vi "Configure Trigger (State).vi"(0 "VISA resource name":refnum<visa-resource-name>, 1 "State Condition (0: AND)":i32(ring) items=["And", "Not And"], 5 "Trigger Source (1: Channel1)":i32(ring)=1 items=["Channel1"=1, "Channel2"=2, "Channel3"=3, "Channel4"=4, "DIG0"=20, "DIG1"=21, "DIG2"=22, "DIG3"=23, "DIG4"=24, "DIG5"=25, "DIG6"=26, "DIG7"=27, "DIG8"=28, "DIG9"=29, "DIG10"=30, "DIG11"=31, "DIG12"=32, "DIG13"=33, "DIG14"=34, "DIG15"=35], 7 "Logic State (0: Low)":i32(ring) items=["Low", "High", "Don't Care"], 9 "State Trigger Slope (0: Rise)":i32(ring) items=["Rising", "Falling", "Either"], 11 "error in (no error)":errorcluster) -> (4 "VISA resource name out":refnum<visa-resource-name>, 15 "error out":errorcluster)   [LabVIEW 2020, in "Agilent 90000 Series.lvlib"]
doc: "Configures state trigger parameters."
uses:
  Agilent 90000 Series.lvlib
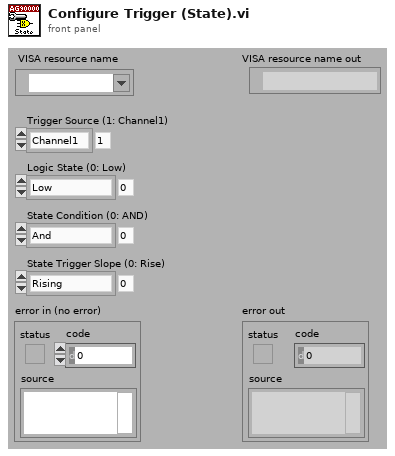
[diagram p1: front panel]
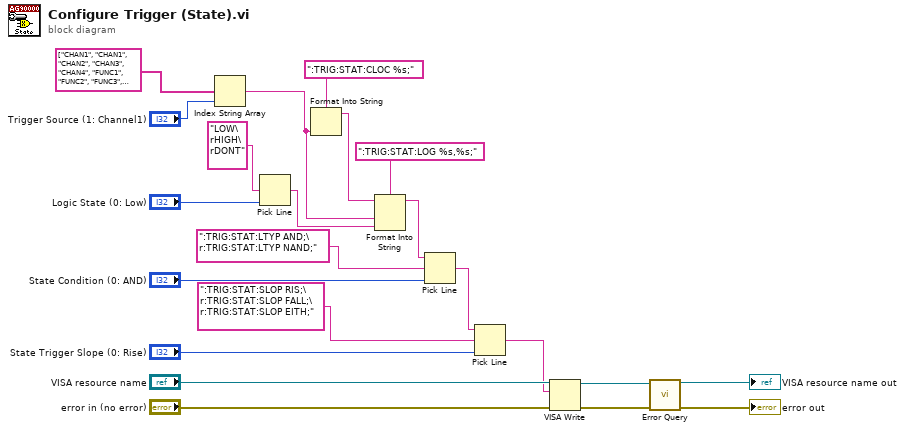
[diagram p0: block diagram]
diagram:
  n1 = Index String Array(1:"Trigger Source (1: Channel1)", 2:string[] ["CHAN1", "CHAN1", "CHAN2", "CHAN3", "CHAN4", "FUNC1", "FUNC2", "FUNC3", "FUNC4", "WMEM1", "WMEM2", "WMEM3", "WMEM4", "AUX", "LINE", "", "", "", "", "", "DIG0", "DIG1", "DIG2", "DIG3", "DIG4", "DIG5", "DIG6", "DIG7", "DIG8", "DIG9", "DIG10", "DIG11", "DIG12", "DIG13", "DIG14", "DIG15", "", ""]) -> (0:w7:string)  [unwired: 1 out]
  n2 = Pick Line(multi-line string="LOW\rHIGH\rDONT", line index="Logic State (0: Low)") -> (output string=w19:string)  [unwired: 1 out]
  n3 = Format Into String(format string=":TRIG:STAT:CLOC %s;", w7) -> (resulting string=w5:string)  [unwired: 2 in, 1 out]
  n4 = Format Into String(format string=":TRIG:STAT:LOG %s,%s;", initial string=w5, w7, w19) -> (resulting string=w6:string)  [unwired: 1 in, 1 out]
  n5 = Pick Line(string ("")=w6, multi-line string=":TRIG:STAT:LTYP AND;\r:TRIG:STAT:LTYP NAND;", line index="State Condition (0: AND)") -> (output string=w4:string)
  n6 = Pick Line(string ("")=w4, multi-line string=":TRIG:STAT:SLOP RIS;\r:TRIG:STAT:SLOP FALL;\r:TRIG:STAT:SLOP EITH;", line index="State Trigger Slope (0: Rise)") -> (output string=w3:string)
  n7 = VISA Write(VISA resource name="VISA resource name", write buffer=w3, error in (no error)="error in (no error)") -> (VISA resource name out=w12:refnum<visa-resource-name>, error out=w11:errorcluster)  [unwired: 1 out]
  n8 = call "Error Query.vi"("error in (no error)"=w11, "VISA resource name"=w12) -> ("error out"=→"error out":errorcluster, "VISA resource name out"=→"VISA resource name out":refnum<visa-resource-name>)  [unwired: 8 out]
